vi "shutdown background process.vi"(8 "error in":errorcluster, 11 "asynchronous execution module runtime In":refnum<class "asynchronous execution module runtime.lvclass">) -> (0 "error out":errorcluster, 3 "asynchronous execution module runtime Out":refnum<class "asynchronous execution module runtime.lvclass">)   [LabVIEW 2013, in "asynchronous execution module runtime.lvclass"]
uses:
  asynchronous execution module runtime.lvclass
  asynchronous execution module runtime.lvclass/asynchronous execution module runtime.ctl
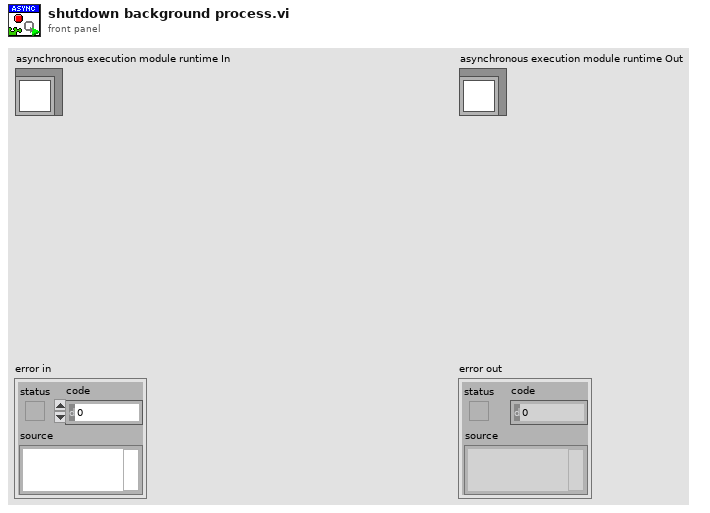
[diagram p1: front panel]
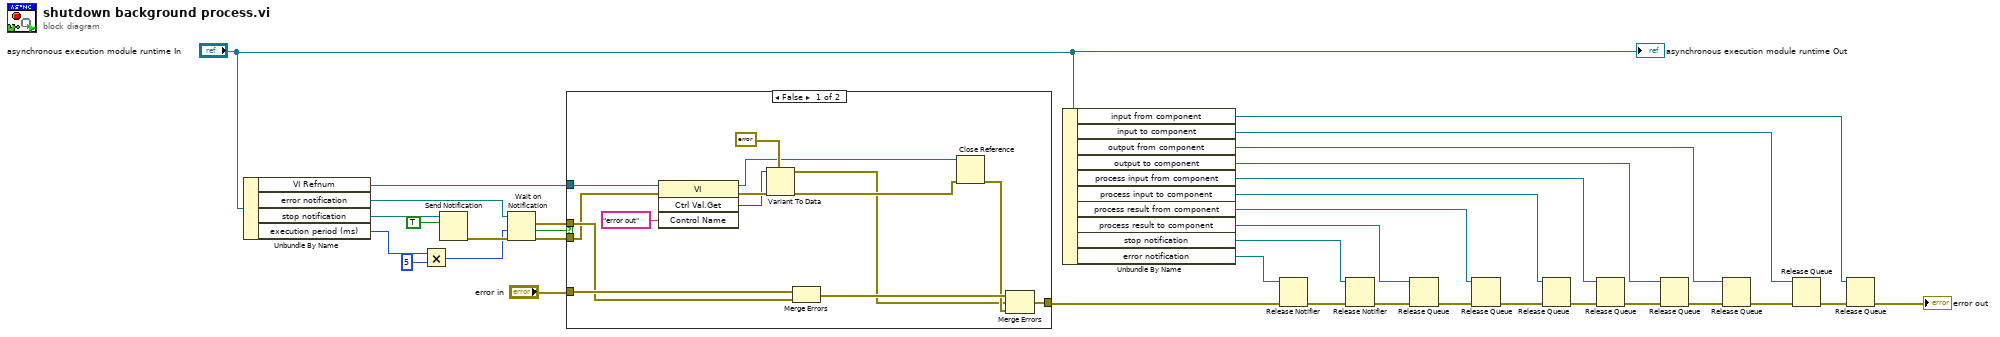
[diagram p0: block diagram]
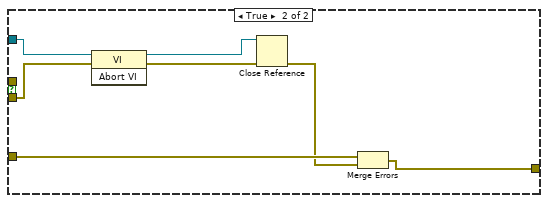
[diagram p2: hidden frame]
diagram:
  n1 = Unbundle By Name("asynchronous execution module runtime In") -> ("VI Refnum"=w4:refnum<vi>, "error notification"=w32:refnum<notifier>, "stop notification"=w34:refnum<notifier>, "execution period (ms)"=w3:i32)
  n2 = Multiply(x=w3, y=5) -> (x*y=w1:i32)
  n3 = Send Notification(notification=TRUE, notifier=w34) -> (error out=w31:errorcluster)  [unwired: 1 in, 1 out]
  n4 = Wait on Notification(notifier=w32, timeout in ms (-1)=w1, error in (no error)=w31) -> (notification=w28:errorcluster, timed out?=w30:bool, error out=w29:errorcluster)  [unwired: 1 in, 1 out]
  n5 = case shown="False" w30 {
    tunnel: w29 -> [w41 w55]
    tunnel: w28 -> [w47 _]
    tunnel: "error in" -> [w48 w54]
    tunnel: [w44 w52] -> w26
    tunnel: w4 -> [w43 w50]
    frame False {
      n6 = invoke class="VI" method="Ctrl Val.Get"(reference=w43, error in=w41, "Control Name"="error out") -> (reference out=w37:refnum<vi>, error out=w40:errorcluster, "Get Control Value Variant"=w39:variant)  [unwired: 1 in, 1 out]
      n7 = Variant To Data(error in=w40, type=errorcluster {"status"=FALSE, "code"=0, "source"=""} ("error constant"), Variant=w39) -> (data=w35:errorcluster, error out=w36:errorcluster)
      n8 = Merge Errors(w48, w47) -> (w46:errorcluster)
      n9 = Close Reference(reference=w37, error in (no error)=w36) -> (error out=w45:errorcluster)
      n10 = Merge Errors(w46, w35, w45) -> (w44:errorcluster)
    }
    frame True {
      n11 = invoke class="VI" method="Abort VI"(reference=w50, error in=w55) -> (reference out=w49:refnum<vi>, error out=w51:errorcluster)  [unwired: 1 in, 1 out]
      n12 = Close Reference(reference=w49, error in (no error)=w51) -> (error out=w53:errorcluster)
      n13 = Merge Errors(w54, w53) -> (w52:errorcluster)
    }
  }
  n14 = Unbundle By Name("asynchronous execution module runtime In") -> ("input from component"=w5:refnum<queue>, "input to component"=w6:refnum<queue>, "output from component"=w7:refnum<queue>, "output to component"=w8:refnum<queue>, "process input from component"=w19:refnum<queue>, "process input to component"=w18:refnum<queue>, "process result from component"=w17:refnum<queue>, "process result to component"=w16:refnum<queue>, "stop notification"=w15:refnum<notifier>, "error notification"=w14:refnum<notifier>)
  n15 = Release Notifier(notifier=w14, error in (no error)=w26) -> (error out=w25:errorcluster)  [unwired: 1 in, 2 out]
  n16 = Release Notifier(notifier=w15, error in (no error)=w25) -> (error out=w21:errorcluster)  [unwired: 1 in, 2 out]
  n17 = Release Queue(queue=w16, error in (no error)=w21) -> (error out=w22:errorcluster)  [unwired: 1 in, 2 out]
  n18 = Release Queue(queue=w17, error in (no error)=w22) -> (error out=w23:errorcluster)  [unwired: 1 in, 2 out]
  n19 = Release Queue(queue=w18, error in (no error)=w23) -> (error out=w24:errorcluster)  [unwired: 1 in, 2 out]
  n20 = Release Queue(queue=w19, error in (no error)=w24) -> (error out=w10:errorcluster)  [unwired: 1 in, 2 out]
  n21 = Release Queue(queue=w8, error in (no error)=w10) -> (error out=w13:errorcluster)  [unwired: 1 in, 2 out]
  n22 = Release Queue(queue=w7, error in (no error)=w13) -> (error out=w12:errorcluster)  [unwired: 1 in, 2 out]
  n23 = Release Queue(queue=w6, error in (no error)=w12) -> (error out=w11:errorcluster)  [unwired: 1 in, 2 out]
  n24 = Release Queue(queue=w5, error in (no error)=w11) -> (error out=→"error out":errorcluster)  [unwired: 1 in, 2 out]
  "asynchronous execution module runtime Out" <- "asynchronous execution module runtime In"
